vi "Template_ASCII String To Data.vi"(8 "error in (no error)":errorcluster, 9 "Default":T1, 11 "Value":string) -> (0 "error out":errorcluster, 3 "Data":T1)   [LabVIEW 2016, in "CVT.lvlib" / "Current Value Table.lvlib"]
doc: "This VI converts data stored on disk as an ascii string into the correct data type. This VI must perform the opposite operation to the DataToASCIIString function."
uses:
  <vilib>/NI/Current Value Table/Current Value Table.lvlib
  <vilib>/NI/Current Value Table/DataTypes/Template_Datatype.ctl
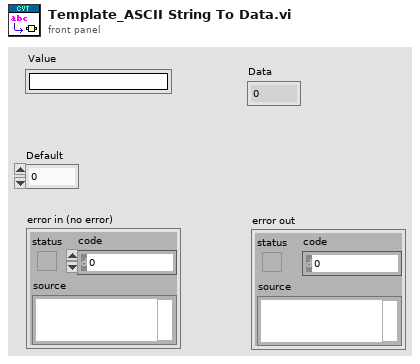
[diagram p1: front panel]
types:
  T1 = typedef "CVT.lvlib/Current Value Table.lvlib/Template_Datatype.ctl" = i32
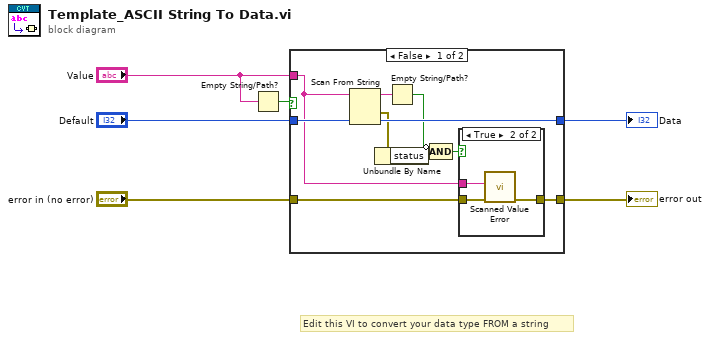
[diagram p0: block diagram]
diagram:
  # "Edit this VI to convert your data type FROM a string"
  n1 = Empty String/Path?(string/path="Value") -> (empty?=w3:bool)
  n2 = case shown="False" w3 {
    tunnel: "Default" -> [w16 w22]
    tunnel: "Value" -> [w8 _]
    tunnel: [w15 w22] -> w1
    tunnel: "error in (no error)" -> [w9 w21]
    tunnel: [w10 w21] -> w5
    frame False {
      n3 = Scan From String(input string=w8, default 1=w16) -> (remaining string=w14:string, error out=w12:errorcluster, output 1=w15:T1)  [unwired: 3 in, 1 out]
      n4 = Unbundle By Name(w12) -> ("status"=w7:bool)
      n5 = Empty String/Path?(string/path=w14) -> (empty?=w13:bool)
      n6 = Compound Arithmetic op=AND(invert w13, w7) -> (w11:bool)
      n7 = case shown="True" w11 {
        tunnel: [w17 w20] -> w10
        tunnel: w9 -> [w17 w19]
        tunnel: w8 -> [_ w18]
        frame False {
        }
        frame True {
          n8 = call <vilib>:"Scanned Value Error.vi"("error in (no error)"=w19, "Value"=w18) -> ("error out"=w20:errorcluster)  [unwired: 9 in]
        }
      }
    }
    frame True {
    }
  }
  "error out" <- w5
  "Data" <- w1
